vi "WriteSamplerate.vi"(8 "Error In":errorcluster, 10 "Samplerate":dbl, 11 "object in":refnum<class "DC Config.lvclass">) -> (0 "Error Out":errorcluster, 3 "object out":refnum<class "DC Config.lvclass">)   [LabVIEW 2023, in "HAL.lvlib" / "PXI-5441.lvlib" / "DC Config.lvclass"]
uses:
  DC Config.lvclass
  DC Config.lvclass/DC Config.ctl
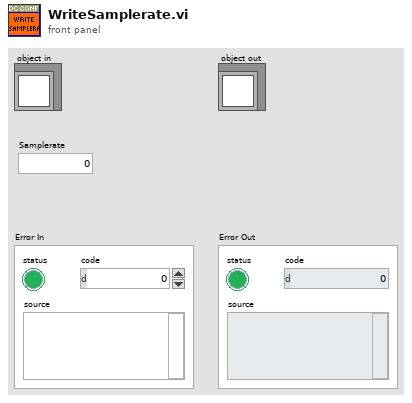
[diagram p1: front panel]
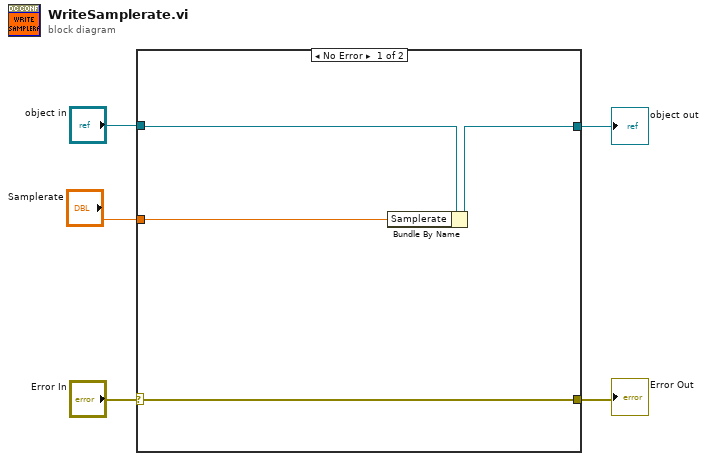
[diagram p0: block diagram]
diagram:
  n1 = case shown="No Error" "Error In" {
    selector: "Error In" -> [w8 w11]
    tunnel: [w8 w11] -> w4
    tunnel: [w6 w10] -> w2
    tunnel: "object in" -> [w7 w10]
    tunnel: "Samplerate" -> [w9 _]
    frame No Error {
      n2 = Bundle By Name(cluster=w7, "Samplerate"=w9) -> (w6:refnum<class "DC Config.lvclass">)
    }
    frame Error {
    }
  }
  "Error Out" <- w4
  "object out" <- w2
